vi "Stepper -- V5.vi"() -> ()   [LabVIEW 2018]
doc: "Use this template to build a producer/consumer design pattern with events to produce queue items. Use this design pattern instead of the User Interface Event Handler pattern for user interfaces when you want to execute code asynchronously in response to an event without slowing the user interface responsiveness."
uses:
  stepper motor state.ctl
  cursor range mode.ctl
  motor type.ctl
  stepper graphics action.ctl
  stepper driver action.ctl
  stepper progress monitor message.ctl
  talkto async routine action.ctl
  stepper graphics internal state.ctl
  stepper graphics internal event.ctl
  publisher action.ctl
  slider action.ctl
  stepper driver -- BLM.vi
  stepper driver -- arduino.vi
  stepper driver -- IMS.vi
panel:
  in  "Tab Control":enum32{"main", "init&stuff", "ignore", "calc"}(tab)
  in  "cur step":dbl(slide) scale=0.0..16500.0 scale format="%#.0f"
  in  "set step !":dbl(slide)=6549.0 min=0.0 max=16000.0 step=1.0 scale=0.0..16500.0
  in  "set angle!":dbl(slide)=-33.45836363636363 scale=-117.31239621859328..107.97695874136122
  in  "Stop!":bool
  in  "Go!":bool
  in  "check!":bool
  in  "stepper state":T1=enum."stopped"
  in  "XY Graph":cluster{dbl[], dbl[]}[](graph)=[{[-0.25028600695262626, -0.18003028570276625, -0.10977456445290623, -0.03951884320304622, 0.030736878046813798, 0.10099259929667381, 0.17124832054653383, 0.24150404179639384, 0.31175976304625386, 0.38201548429611387, 0.4522712055459739, 0.5225269267958339, 0.5927826480456939, 0.6630383692955539, 0.733294090545414, 0.803549811795274, 0.873805533045134, 0.944061254294994, 1.014316975544854, 1.084572696794714], [0.16539925853434134, 0.11897139648961394, 0.07254353444488655, 0.026115672400159162, -0.02031218964456824, -0.06674005168929564, -0.11316791373402302, -0.15959577577875045, -0.20602363782347782, -0.2524514998682052, -0.29887936191293263, -0.34530722395766, -0.3917350860023874, -0.43816294804711475, -0.48459081009184224, -0.5310186721365696, -0.577446534181297, -0.6238743962260244, -0.6703022582707517, -0.7167301203154792]}, {[0.14084146883576712, 0.11119063329139509, 0.08153979774702305, 0.05188896220265103, 0.022238126658278998, -0.007412708886093022, -0.037063544430465056, -0.06671437997483709, -0.09636521551920912, -0.12601605106358113, -0.15566688660795316, -0.1853177221523252, -0.21496855769669723, -0.24461939324106927, -0.2742702287854413, -0.30392106432981336, -0.33357189987418534, -0.36322273541855743, -0.3928735709629294, -0.4225244065073015], [0.26488427785767804, 0.20911916672974581, 0.1533540556018136, 0.09758894447388133, 0.04182383334594911, -0.013941277781983119, -0.06970638890991537, -0.12547150003784757, -0.18123661116577983, -0.23700172229371202, -0.2927668334216443, -0.34853194454957653, -0.4042970556775088, -0.46006216680544104, -0.5158272779333732, -0.5715923890613055, -0.6273575001892377, -0.68312261131717, -0.738887722445102, -0.7946528335730343]}, {[1.0, 0.9980267284282716, 0.9921147013144779, 0.9822872507286887, 0.9685831611286311, 0.9510565162951535, 0.9297764858882513, 0.9048270524660195, 0.8763066800438636, 0.8443279255020151, 0.8090169943749475, 0.7705132427757891, 0.7289686274214116, 0.6845471059286886, 0.6374239897486896, 0.587785252292473, 0.5358267949789965, 0.48175367410171516, 0.42577929156507266, 0.36812455268467786, 0.30901699437494745, 0.24868988716485474, 0.18738131458572452, 0.12533323356430426, 0.0627905195293133, -1.6081428723391245e-16, -0.0627905195293134, -0.12533323356430437, -0.18738131458572482, -0.24868988716485485, -0.30901699437494756, -0.368124552684678, -0.4257792915650727, -0.48175367410171543, -0.5358267949789969, -0.587785252292473, -0.6374239897486897, -0.6845471059286887, -0.7289686274214117, -0.7705132427757894, -0.8090169943749473, -0.8443279255020151, -0.8763066800438636, -0.9048270524660196, -0.9297764858882515, -0.9510565162951536, -0.9685831611286311, -0.9822872507286887, -0.9921147013144779, -0.9980267284282716, -1.0, -0.9980267284282716, -0.9921147013144779, -0.9822872507286886, -0.9685831611286311, -0.9510565162951535, -0.9297764858882512, -0.9048270524660195, -0.8763066800438635, -0.844327925502015, -0.8090169943749472, -0.770513242775789, -0.7289686274214116, -0.6845471059286886, -0.6374239897486895, -0.5877852522924732, -0.5358267949789963, -0.48175367410171527, -0.42577929156507216, -0.3681245526846778, -0.30901699437494756, -0.24868988716485443, -0.18738131458572463, -0.12533323356430373, -0.06279051952931321, -1.836909530733566e-16, 0.06279051952931372, 0.12533323356430423, 0.18738131458572513, 0.24868988716485493, 0.30901699437494723, 0.36812455268467825, 0.4257792915650726, 0.4817536741017157, 0.5358267949789968, 0.5877852522924737, 0.63742398974869, 0.6845471059286886, 0.7289686274214119, 0.7705132427757894, 0.8090169943749478, 0.8443279255020153, 0.8763066800438636, 0.9048270524660197, 0.9297764858882515, 0.9510565162951538, 0.9685831611286312, 0.9822872507286887, 0.9921147013144779, 0.9980267284282716], [0.0, 0.06279051952931337, 0.12533323356430426, 0.18738131458572463, 0.2486898871648548, 0.3090169943749474, 0.368124552684678, 0.4257792915650727, 0.4817536741017153, 0.5358267949789967, 0.5877852522924731, 0.6374239897486897, 0.6845471059286887, 0.7289686274214116, 0.7705132427757893, 0.8090169943749475, 0.8443279255020151, 0.8763066800438637, 0.9048270524660196, 0.9297764858882515, 0.9510565162951535, 0.9685831611286311, 0.9822872507286887, 0.9921147013144779, 0.9980267284282716, 1.0, 0.9980267284282716, 0.9921147013144778, 0.9822872507286886, 0.9685831611286311, 0.9510565162951535, 0.9297764858882513, 0.9048270524660195, 0.8763066800438635, 0.844327925502015, 0.8090169943749475, 0.7705132427757893, 0.7289686274214114, 0.6845471059286885, 0.6374239897486895, 0.5877852522924732, 0.5358267949789967, 0.4817536741017152, 0.4257792915650725, 0.36812455268467775, 0.3090169943749471, 0.24868988716485482, 0.18738131458572457, 0.1253332335643041, 0.06279051952931314, -3.216285744678249e-16, -0.06279051952931335, -0.12533323356430429, -0.18738131458572477, -0.24868988716485502, -0.30901699437494773, -0.3681245526846783, -0.42577929156507266, -0.4817536741017154, -0.5358267949789968, -0.5877852522924734, -0.63742398974869, -0.6845471059286887, -0.7289686274214116, -0.7705132427757894, -0.8090169943749473, -0.8443279255020153, -0.8763066800438636, -0.9048270524660198, -0.9297764858882515, -0.9510565162951535, -0.9685831611286312, -0.9822872507286887, -0.9921147013144779, -0.9980267284282716, -1.0, -0.9980267284282716, -0.9921147013144779, -0.9822872507286886, -0.9685831611286311, -0.9510565162951536, -0.9297764858882512, -0.9048270524660196, -0.8763066800438634, -0.844327925502015, -0.809016994374947, -0.770513242775789, -0.7289686274214116, -0.6845471059286883, -0.6374239897486896, -0.5877852522924726, -0.5358267949789963, -0.4817536741017153, -0.4257792915650722, -0.36812455268467786, -0.3090169943749468, -0.2486898871648545, -0.18738131458572468, -0.1253332335643038, -0.06279051952931326]}, {[0.1, 0.09980267284282716, 0.0992114701314478, 0.09822872507286887, 0.09685831611286312, 0.09510565162951537, 0.09297764858882515, 0.09048270524660196, 0.08763066800438636, 0.08443279255020152, 0.08090169943749474, 0.07705132427757892, 0.07289686274214115, 0.06845471059286887, 0.06374239897486897, 0.05877852522924731, 0.05358267949789966, 0.04817536741017152, 0.042577929156507266, 0.03681245526846779, 0.03090169943749475, 0.024868988716485477, 0.018738131458572452, 0.012533323356430426, 0.00627905195293133, -1.6081428723391246e-17, -0.0062790519529313405, -0.012533323356430436, -0.018738131458572484, -0.024868988716485487, -0.030901699437494757, -0.0368124552684678, -0.04257792915650727, -0.048175367410171546, -0.05358267949789969, -0.05877852522924731, -0.06374239897486897, -0.06845471059286888, -0.07289686274214117, -0.07705132427757895, -0.08090169943749474, -0.08443279255020152, -0.08763066800438636, -0.09048270524660197, -0.09297764858882515, -0.09510565162951537, -0.09685831611286312, -0.09822872507286888, -0.0992114701314478, -0.09980267284282716, -0.1, -0.09980267284282716, -0.0992114701314478, -0.09822872507286887, -0.09685831611286311, -0.09510565162951536, -0.09297764858882514, -0.09048270524660196, -0.08763066800438636, -0.0844327925502015, -0.08090169943749473, -0.07705132427757891, -0.07289686274214116, -0.06845471059286887, -0.06374239897486896, -0.05877852522924733, -0.05358267949789963, -0.04817536741017153, -0.04257792915650722, -0.036812455268467784, -0.03090169943749476, -0.024868988716485445, -0.018738131458572463, -0.012533323356430372, -0.0062790519529313206, -1.836909530733566e-17, 0.006279051952931373, 0.012533323356430424, 0.018738131458572515, 0.024868988716485498, 0.030901699437494726, 0.03681245526846783, 0.042577929156507266, 0.048175367410171574, 0.053582679497899674, 0.05877852522924737, 0.063742398974869, 0.06845471059286887, 0.07289686274214119, 0.07705132427757894, 0.08090169943749478, 0.08443279255020153, 0.08763066800438636, 0.09048270524660197, 0.09297764858882515, 0.09510565162951538, 0.09685831611286312, 0.09822872507286887, 0.0992114701314478, 0.09980267284282716], [0.0, 0.006279051952931338, 0.012533323356430426, 0.018738131458572466, 0.02486898871648548, 0.030901699437494743, 0.0368124552684678, 0.04257792915650727, 0.04817536741017153, 0.05358267949789967, 0.058778525229247314, 0.06374239897486898, 0.06845471059286887, 0.07289686274214116, 0.07705132427757894, 0.08090169943749476, 0.08443279255020152, 0.08763066800438638, 0.09048270524660196, 0.09297764858882515, 0.09510565162951536, 0.09685831611286312, 0.09822872507286888, 0.0992114701314478, 0.09980267284282716, 0.1, 0.09980267284282716, 0.0992114701314478, 0.09822872507286887, 0.09685831611286312, 0.09510565162951536, 0.09297764858882515, 0.09048270524660196, 0.08763066800438636, 0.0844327925502015, 0.08090169943749476, 0.07705132427757892, 0.07289686274214115, 0.06845471059286885, 0.06374239897486896, 0.05877852522924732, 0.05358267949789967, 0.048175367410171525, 0.04257792915650725, 0.03681245526846778, 0.030901699437494712, 0.024868988716485484, 0.01873813145857246, 0.01253332335643041, 0.0062790519529313145, -3.216285744678249e-17, -0.0062790519529313344, -0.012533323356430431, -0.018738131458572477, -0.0248689887164855, -0.030901699437494774, -0.03681245526846783, -0.04257792915650727, -0.04817536741017154, -0.05358267949789968, -0.05877852522924734, -0.06374239897486901, -0.06845471059286887, -0.07289686274214116, -0.07705132427757894, -0.08090169943749474, -0.08443279255020153, -0.08763066800438636, -0.09048270524660199, -0.09297764858882515, -0.09510565162951536, -0.09685831611286312, -0.09822872507286888, -0.0992114701314478, -0.09980267284282716, -0.1, -0.09980267284282716, -0.0992114701314478, -0.09822872507286887, -0.09685831611286311, -0.09510565162951537, -0.09297764858882514, -0.09048270524660196, -0.08763066800438633, -0.0844327925502015, -0.0809016994374947, -0.07705132427757891, -0.07289686274214116, -0.06845471059286884, -0.06374239897486897, -0.058778525229247265, -0.05358267949789964, -0.04817536741017153, -0.042577929156507224, -0.036812455268467784, -0.03090169943749468, -0.024868988716485452, -0.01873813145857247, -0.012533323356430379, -0.006279051952931327]}, {[-1.7, -1.7, -1.7, -1.7, -1.7, -1.7, -1.7, -1.7, -1.7, -1.7, -1.7, -1.7, -1.7, -1.7, -1.7, -1.7, -1.7, -1.7, -1.7, -1.7, -1.7, -1.6105263157894736, -1.5210526315789474, -1.431578947368421, -1.3421052631578947, -1.2526315789473683, -1.163157894736842, -1.0736842105263158, -0.9842105263157894, -0.894736842105263, -0.8052631578947368, -0.7157894736842105, -0.6263157894736842, -0.5368421052631578, -0.44736842105263164, -0.35789473684210527, -0.2684210526315789, -0.17894736842105252, -0.08947368421052615, 0.0, 0.0, 0.08947368421052632, 0.17894736842105263, 0.26842105263157895, 0.35789473684210527, 0.4473684210526316, 0.5368421052631579, 0.6263157894736842, 0.7157894736842105, 0.8052631578947369, 0.8947368421052632, 0.9842105263157894, 1.0736842105263158, 1.1631578947368422, 1.2526315789473683, 1.3421052631578947, 1.431578947368421, 1.5210526315789474, 1.6105263157894738, 1.7, 1.7, 1.7, 1.7, 1.7, 1.7, 1.7, 1.7, 1.7, 1.7, 1.7, 1.7, 1.7, 1.7, 1.7, 1.7, 1.7, 1.7, 1.7, 1.7, 1.7], [1.9, 1.7210526315789472, 1.5421052631578946, 1.3631578947368421, 1.1842105263157894, 1.0052631578947366, 0.8263157894736841, 0.6473684210526316, 0.46842105263157885, 0.2894736842105261, 0.11052631578947358, -0.06842105263157894, -0.24736842105263168, -0.4263157894736844, -0.6052631578947367, -0.7842105263157895, -0.9631578947368422, -1.142105263157895, -1.3210526315789477, -1.5, -1.5, -1.5257894736842106, -1.551578947368421, -1.5773684210526315, -1.6031578947368421, -1.6289473684210527, -1.654736842105263, -1.6805263157894736, -1.7063157894736842, -1.7321052631578948, -1.7578947368421052, -1.7836842105263158, -1.8094736842105263, -1.8352631578947367, -1.8610526315789473, -1.8868421052631579, -1.9126315789473685, -1.938421052631579, -1.9642105263157894, -1.99, -1.9900000000000002, -1.9642105263157896, -1.9384210526315793, -1.9126315789473687, -1.886842105263158, -1.8610526315789475, -1.8352631578947372, -1.8094736842105266, -1.783684210526316, -1.7578947368421054, -1.732105263157895, -1.7063157894736845, -1.6805263157894739, -1.6547368421052635, -1.628947368421053, -1.6031578947368423, -1.5773684210526318, -1.5515789473684212, -1.5257894736842108, -1.5000000000000002, -1.5, -1.3210526315789473, -1.1421052631578947, -0.9631578947368421, -0.7842105263157895, -0.6052631578947368, -0.4263157894736842, -0.24736842105263168, -0.06842105263157894, 0.1105263157894738, 0.2894736842105263, 0.46842105263157885, 0.6473684210526316, 0.8263157894736843, 1.0052631578947366, 1.1842105263157894, 1.3631578947368421, 1.5421052631578949, 1.7210526315789476, 1.9]}, {[-0.08715574274765822, -0.08899060048971419, -0.09082545823177014, -0.09266031597382611, -0.09449517371588206, -0.09633003145793803, -0.098164889199994, -0.09999974694204995, -0.10183460468410592, -0.10366946242616187, -0.10550432016821784, -0.10733917791027381, -0.10917403565232978, -0.11100889339438573, -0.1128437511364417, -0.11467860887849765, -0.11651346662055362, -0.11834832436260959, -0.12018318210466554, -0.12201803984672151], [0.9961946980917454, 1.0171672180515716, 1.038139738011398, 1.059112257971224, 1.0800847779310503, 1.1010572978908766, 1.1220298178507027, 1.143002337810529, 1.1639748577703553, 1.1849473777301813, 1.2059198976900076, 1.2268924176498337, 1.24786493760966, 1.2688374575694863, 1.2898099775293124, 1.3107824974891387, 1.3317550174489647, 1.352727537408791, 1.3737000573686173, 1.3946725773284436]}, {[-0.46947156278589053, -0.47935517463401456, -0.48923878648213853, -0.49912239833026256, -0.5090060101783865, -0.5188896220265106, -0.5287732338746346, -0.5386568457227586, -0.5485404575708825, -0.5584240694190066, -0.5683076812671306, -0.5781912931152546, -0.5880749049633787, -0.5979585168115026, -0.6078421286596266, -0.6177257405077506, -0.6276093523558747, -0.6374929642039986, -0.6473765760521226, -0.6572601879002467], [-0.882947592858927, -0.9015359632349044, -0.9201243336108818, -0.9387127039868592, -0.9573010743628366, -0.975889444738814, -0.9944778151147914, -1.0130661854907688, -1.0316545558667463, -1.0502429262427238, -1.068831296618701, -1.0874196669946785, -1.1060080373706558, -1.1245964077466333, -1.1431847781226105, -1.161773148498588, -1.1803615188745655, -1.1989498892505428, -1.2175382596265203, -1.2361266300024978]}, {[-0.6572601879002467, -0.6108630096264345, -0.5636217044296241, -0.515601553161604, -0.46686891293009347, -0.41749112540253713, -0.3675364237493727, -0.31707383835536895, -0.26617310142932604, -0.21490455064395006, -0.1633390319390661, -0.11154780162247316, -0.05960242790373095, -0.007574691996942432, 0.044463511070809286, 0.09644027180829284, 0.1482837656289526, 0.19992235210240325, 0.25128467395144666, 0.3022997556578122, 0.35289710154035936, 0.4030067931702119, 0.45255958598821155, 0.5014870049911768, 0.5497214393547454, 0.5971962358620418, 0.643845791009066, 0.6896056416595259, 0.7344125541238411, 0.7782046115392272, 0.8209212994301052, 0.8625035893306137, 0.9028940203536602, 0.9420367785938017, 0.979877774254226, 1.0163647163912568, 1.0514471851730987, 1.0850767015529643, 1.1172067942603134, 1.1477930640176235, 1.176793244893958, 1.204167262710551, 1.2298772904176951, 1.2538878003664136, 1.276165613402685, 1.2966799447163748, 1.3154024463815224, 1.3323072465291936, 1.3473709850987734, 1.360572846118289, 1.3718945864691614, 1.3813205610956336, 1.3888377446240419, 1.3944357493620536, 1.3981068396529994, 1.3998459425654655, 1.399650654903371, 1.3975212465268496, 1.3934606599793398, 1.3874745064214027, 1.379571057876886, 1.3697612358021491, 1.3580585959941422, 1.3444793098581995, 1.3290421420614258, 1.3117684246025616, 1.2926820273341562, 1.2718093249777804, 1.249179160677867, 1.2248228061445314, 1.1987739184404593, 1.1710684934715725, 1.141744816245737, 1.1108434079682614, 1.078406970047275, 1.0444803250863792, 1.0091103549461014, 0.9723459359597438, 0.9342378713931556, 0.894838821241748, 0.8542032294617747, 0.8123872487364283, 0.7694486628807135, 0.7254468069923291, 0.6804424854588903, 0.6344978879348022, 0.5876765034038882, 0.5400430324465261, 0.49166329783253176, 0.4426041535633281, 0.39293339248910303, 0.34271965262860676, 0.2920323223210451, 0.24094144434113837, 0.18951761910983606, 0.1378319071344487, 0.08595573081300137, 0.033960775738508885, -0.018081108360453915, -0.07009800690598791], [-1.2361266300024978, -1.259700910323611, -1.2815344608303927, -1.301597110621156, -1.319861135930395, -1.3363012984391367, -1.3508948801507545, -1.3636217147840501, -1.374464215640223, -1.38340739990522, -1.3904389093538805, -1.3955490274272677, -1.3987306926595915, -1.3999795084361597, -1.399293749068885, -1.3966743621809423, -1.392124967397287, -1.3856518513428409, -1.3772639589552595, -1.3669728811242843, -1.3547928386747596, -1.3407406627154492, -1.3248357713808072, -1.307100142997842, -1.2875582857151542, -1.266237203636115, -1.243166359502987, -1.2183776339835501, -1.1919052816164948, -1.1637858834764583, -1.1340582966241142, -1.1027636004111705, -1.0699450397144725, -1.0356479651776527, -0.999919770542909, -0.962809827159507, -0.9243694157595043, -0.8846516555949799, -0.8437114310346835, -0.8016053157215436, -0.7583914943958356, -0.7141296824920375, -0.6688810436204844, -0.6227081050478439, -0.5756746712932125, -0.5278457359592277, -0.47928739192003167, -0.4300667399902001, -0.3802517962008339, -0.3299113978109549, -0.279115108184076, -0.22793312066139887, -0.17643616156447195, -0.12469539246134045, -0.07278231183125206, -0.020768656263793716, 0.0312736986710031, 0.08327283774461088, 0.1351569054467535, 0.18685420527963775, 0.23829329883244557, 0.2894031044991896, 0.3401129957035144, 0.39035289849470745, 0.44005338838006564, 0.48914578625979516, 0.5375622533318869, 0.5852358848358173, 0.6321008025055334, 0.6780922456039706, 0.7231466604132986, 0.7672017880572369, 0.8101967505340834, 0.8520721348415629, 0.8927700750772594, 0.9322343324011679, 0.970410372749876, 1.0072454421949844, 1.0426886398416284, 1.0766909881663722, 1.1092055006972668, 1.140187246942561, 1.1695934144783315, 1.1973833681092427, 1.2235187060206834, 1.2479633128446825, 1.2706834095662773, 1.2916476002013708, 1.310826915181573, 1.3281948513860795, 1.3437274087652615, 1.3574031235053672, 1.3692030976884975, 1.3791110254068764, 1.3871132152953265, 1.3931986094508135, 1.3973587987129157, 1.3995880342841027, 1.3998832356737676, 1.398243994955032]}]
  in  "motor selector":T2=enum."--"
  in  "Instrument Address":refnum<visa-resource-name>="ASRL3::INSTR"
  in  "set speed!":bool
  in  "speed":dbl=2.0 format="%_2f"
  in  "sync to":bool
  in  "syncto":dbl format="%_2f"
  in  "cursor mode":T3
  in  "response message":cluster{"step (fdeg)":dbl}={"step (fdeg)"=310.3875004849805}
  out "progress monitor VI":refnum<vi>
  out "cur angle":dbl(slide)=-118.0 scale=-117.31239621859328..107.97695874136122 scale format="%#.0f"
  in  "angle aux":dbl(slide)=86.23585875899897 scale=0.0..90.0 scale format="%#.0f"
  in  "step aux":dbl(slide)=16500.0 scale=0.0..8886.0 scale format="%#.0f"
  in  "dir":u16(ring)
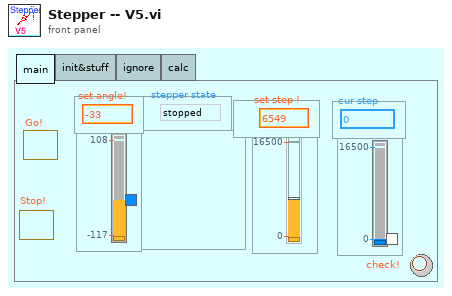
[diagram p1: front panel]
types:
  T1 = typedef "stepper motor state.ctl" = enum16{"moving", "stopped"}
  T2 = typedef "motor type.ctl" = enum16{"IMS", "arduino C&A", "BLM", "--"}
  T3 = typedef "cursor range mode.ctl" = enum16{"change angle", "lock", "extend"}
  T4 = typedef "stepper graphics action.ctl" = enum16{"--update circle", "set step slider moves", "cursor moves", "current step changed", "init", "void", "--draw current line", "--draw set line", "--move current step slider", "--move set step slider", "--draw limit lines", "check", "--move set angle slider", "--move current angle slider", "set angle slider moves", "--move center cursor", "set set step", "set current step", "read", "--move limit-cursors", "cursor release", "current step moves"}
  T5 = typedef "stepper driver action.ctl" = enum16{"go", "void", "stop", "check", "init", "sync", "set", "set speed", "--check status", "--check value", "--handshake"}
  T6 = typedef "stepper graphics internal event.ctl" = enum16{"set slider moves", "update scale", "exit", "current positon changed", "stop", "go", "set speed", "set to zero", "sync", "check"}
  T7 = typedef "stepper graphics internal state.ctl" = cluster{"set pos slider":refnum<vi>, "cur angle slider":refnum<vi>, "XY Graph":refnum<vi>, "set angle":dbl, "current angle":dbl, "set angle slider":refnum<vi>, "current pos... slider":refnum<vi>, "current pos":dbl, "set pos":dbl}
  T8 = typedef "talkto async routine action.ctl" = enum16{"stop", "check"}
  T9 = typedef "stepper progress monitor message.ctl" = cluster{"current position":dbl, "stepper motor state OUT":T1}
  T10 = typedef "publisher action.ctl" = enum16{"set", "get", "init", "check"}
  T11 = typedef "slider action.ctl" = enum16{"check", "copy range -- keep value", "set from value", "set from ratio", "set from slider", "read using other slider", "set lower limit", "set upper limit", "set lower from slider", "set upper from slider", "copy range -- keep ratio", "set using other slider -- no check"}
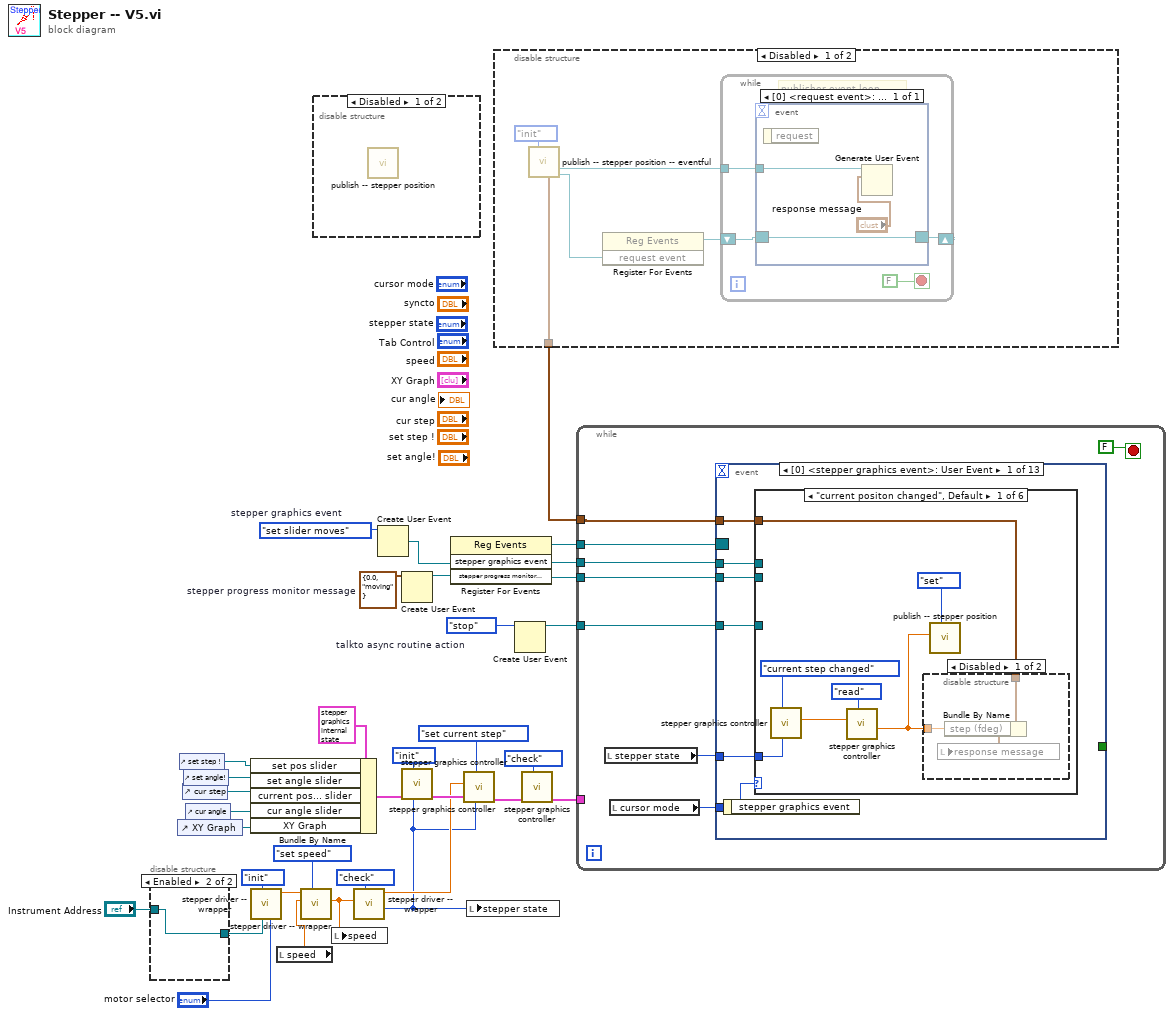
[diagram p0: block diagram]
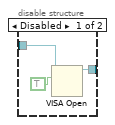
[diagram p2: hidden frame]
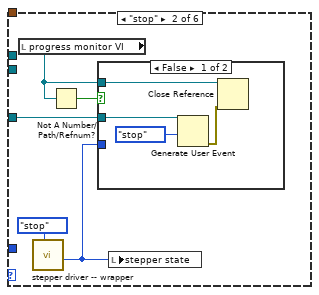
[diagram p6: hidden frame]
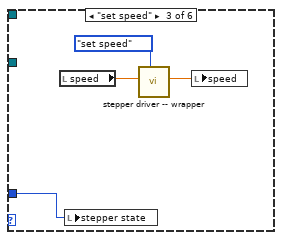
[diagram p8: hidden frame]
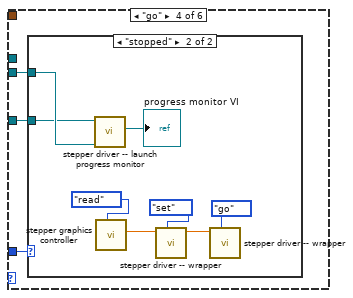
[diagram p9: hidden frame]
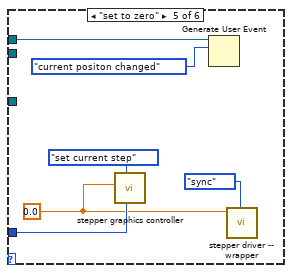
[diagram p11: hidden frame]
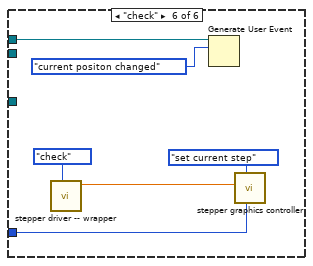
[diagram p12: hidden frame]
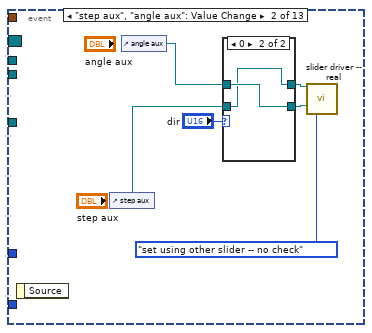
[diagram p13: hidden frame]
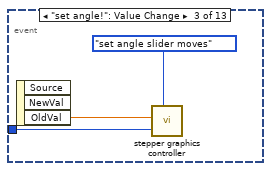
[diagram p15: hidden frame]
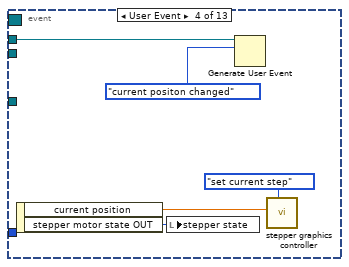
[diagram p16: hidden frame]
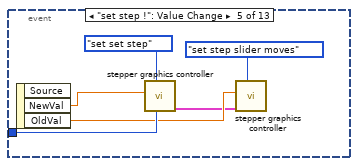
[diagram p17: hidden frame]
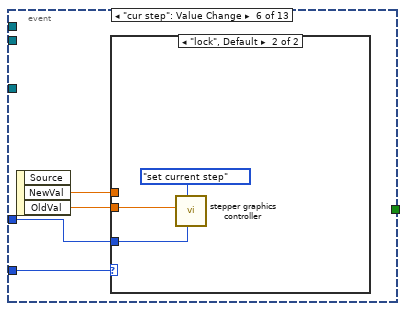
[diagram p18: hidden frame]
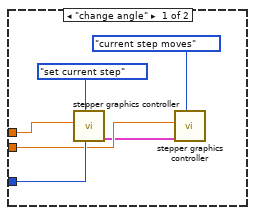
[diagram p19: hidden frame]
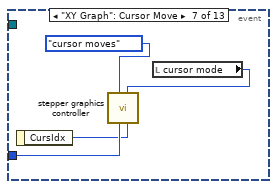
[diagram p20: hidden frame]
diagram:
  w15 = stepper_graphics_internal_event."set slider moves"  # stepper graphics event
  w25 = talkto_async_routine_action."stop"  # talkto async routine action
  w27 = T9 {"current position"=0.0, "stepper motor state OUT"=enum."moving"}  # stepper progress monitor message
  n1 = disable-structure shown="Enabled" {
    disable-tunnel: "Instrument Address" -> [w34 w36]
    disable-tunnel: [w33 w36] -> w14
    frame Disabled {
      n2 = VISA Open(duplicate session (F)=TRUE, VISA resource name=w34) -> (VISA resource name=w33:refnum<visa-resource-name>)  [unwired: 3 in, 1 out]
    }
    frame Enabled {
    }
  }
  n3 = control-ref of="XY Graph"() -> (w18:refnum<vi>)
  n4 = control-ref of="set step !"() -> (w22:refnum<vi>)
  n5 = control-ref of="cur step"() -> (w20:refnum<vi>)
  n6 = control-ref of="set angle!"() -> (w21:refnum<vi>)
  n7 = control-ref of="cur angle"() -> (w19:refnum<vi>)
  n8 = Bundle By Name(cluster=T7 {"set pos slider"=refnum, "cur angle slider"=refnum, "XY Graph"=refnum, "set angle"=0.0, "current angle"=0.0, "set angle slider"=refnum, "current pos... slider"=refnum, "current pos"=0.0, "set pos"=0.0} ("stepper graphics internal state"), "set pos slider"=w22, "set angle slider"=w21, "current pos... slider"=w20, "cur angle slider"=w19, "XY Graph"=w18) -> (w16:T7)
  n9 = call "stepper driver -- wrapper.vi"("motor selector"="motor selector", "Instrument Address"=w14, "stepper driver action"=stepper_driver_action."init") -> ("number OUT"=w12:dbl)  [unwired: 6 in, 2 out]
  n10 = local read "speed"() -> (w13:dbl)
  n11 = call "stepper driver -- wrapper.vi"("stepper driver action"=stepper_driver_action."set speed", "speed IN"=w13, "number IN"=w12) -> ("speed OUT"=w6:dbl)  [unwired: 6 in, 2 out]
  n12 = disable-structure shown="Disabled" {
    frame Disabled {
      n13 = call "publish -- stepper position.vi"() -> ()  [unwired: 11 in, 1 out]
    }
    frame Enabled {
    }
  }
  n14 = local write "speed"(w6) -> ()
  n15 = call "stepper driver -- wrapper.vi"("stepper driver action"=stepper_driver_action."check", "speed IN"=w6) -> ("stepper motor state OUT"=w5:T1, "number OUT"=w7:dbl)  [unwired: 7 in, 1 out]
  n16 = Create User Event(user event datatype=w15) -> (user event=w28:refnum<user-event>)  [unwired: 1 in, 1 out]
  n17 = Create User Event(user event datatype=w27) -> (user event=w26:refnum<user-event>)  [unwired: 1 in, 1 out]
  n18 = call "stepper graphics controller.vi"("stepper motor state"=w5, "stepper graphics action"=stepper_graphics_action."init", "stepper graphics internal state"=w16) -> ("stepper graphics internal state OUT"=w8:T7)  [unwired: 6 in, 2 out]
  n19 = register-events(w28, w26) -> (reference out=w31:refnum<event-registration>)  [unwired: 2 in, 1 out]
  n20 = call "stepper graphics controller.vi"("stepper motor state"=w5, "stepper graphics action"=stepper_graphics_action."set current step", "stepper graphics internal state"=w8, "value"=w7) -> ("stepper graphics internal state OUT"=w3:T7)  [unwired: 5 in, 2 out]
  n21 = local write "stepper state"(w5) -> ()
  n22 = disable-structure shown="Disabled" {
    disable-tunnel: [w37 _] -> w11
    frame Disabled {
      n23 = call "publish -- stepper position -- eventful.vi"("publisher action"=publisher_action."init") -> ("response event"=w38:refnum<user-event>, "response type"=w37:cluster{"step (fdeg)":dbl}, "request event"=w39:refnum<user-event>)  [unwired: 11 in, 1 out]
      n24 = register-events(w39) -> (reference out=w40:refnum<event-registration>)  [unwired: 2 in, 1 out]
      n25 = while {
        shift-right: [w44] -> _
        shift-left: w40 -> [w43]
        tunnel: w38 -> [w42]
        stop <- FALSE stop-if-true
        # "publisher event loop"
        n26 = event shown="[0] <request event>: User Event" {
          selector: w43 -> [w48]
          dyn-events: [w48] -> w44
          timeout: _ -> [_]
          tunnel: w42 -> [w47]
          event User Event {
            n27 = event-data() -> ()  [unwired: 1 in, 1 out]
            n28 = Generate User Event(user event=w47, event data cluster="response message") -> ()  [unwired: 2 in, 2 out]
          }
        }
      }
    }
    frame Enabled {
    }
  }
  n29 = Create User Event(user event datatype=w25) -> (user event=w24:refnum<user-event>)  [unwired: 1 in, 1 out]
  n30 = call "stepper graphics controller.vi"("stepper graphics action"=stepper_graphics_action."check", "stepper graphics internal state"=w3) -> ("stepper graphics internal state OUT"=w2:T7)  [unwired: 7 in, 2 out]
  n31 = while {
    tunnel: w31 -> [w56]
    tunnel: w28 -> [w55]
    tunnel: w26 -> [w53]
    tunnel: w24 -> [w52]
    tunnel: w11 -> [w50]
    tunnel: w2 -> [_]
    stop <- FALSE stop-if-true
    n32 = local read "stepper state"() -> (w54:T1)
    n33 = local read "cursor mode"() -> (w49:T3)
    n34 = event shown="[0] <stepper graphics event>: User Event" {
      selector: w56 -> [_ _ _ _ _ _ _ _ _ _ _ _ _]
      dyn-events: _ -> [_ _ _ _ _ _ _ _ _ _ _ _ _]
      timeout: _ -> [_ _ _ _ _ _ _ _ _ _ _ _ _]
      tunnel: w55 -> [w60 _ _ w123 _ _ _ _ w154 w158 w161 w164 w167]
      tunnel: w54 -> [w61 _ w119 _ w131 w136 w148 w151 _ _ _ _ _]
      tunnel: [_ _ _ _ _ _ _ _ "Stop!" "set speed!" "Go!" "check!" "sync to"] -> _
      tunnel: w53 -> [w59 _ _ _ _ _ _ _ _ _ _ _ _]
      tunnel: w52 -> [w58 _ _ _ _ _ _ _ _ _ _ _ _]
      tunnel: w50 -> [w57 _ _ _ _ _ _ _ _ _ _ _ _]
      tunnel: w49 -> [_ _ _ _ _ w133 _ _ _ _ _ _ _]
      event User Event {
        n35 = event-data() -> ("stepper graphics event"=w62:T6)  [unwired: 1 in]
        n36 = case shown="\"current positon changed\", Default" w62 {
          tunnel: w61 -> [w68 _ w82 w87 w101 w107]
          tunnel: w60 -> [_ _ _ _ w99 w105]
          tunnel: w59 -> [_ _ _ w88 _ _]
          tunnel: w58 -> [_ w74 _ w86 _ _]
          tunnel: w57 -> [w65 _ _ _ _ _]
          frame "current positon changed", Default {
            n37 = call "stepper graphics controller.vi"("stepper motor state"=w68, "stepper graphics action"=stepper_graphics_action."current step changed") -> ("set pos"=w66:dbl)  [unwired: 7 in, 2 out]
            n38 = call "stepper graphics controller.vi"("stepper graphics action"=stepper_graphics_action."read", "value"=w66) -> ("current pos"=w64:dbl)  [unwired: 7 in, 2 out]
            n39 = disable-structure shown="Disabled" {
              disable-tunnel: w64 -> [w72 _]
              disable-tunnel: w65 -> [w70 _]
              frame Disabled {
                n40 = Bundle By Name(cluster=w70, "step (fdeg)"=w72) -> (w71:cluster{"step (fdeg)":dbl})
                n41 = local write "response message"(w71) -> ()
              }
              frame Enabled {
              }
            }
            n42 = call "publish -- stepper position.vi"("publisher action"=publisher_action."set", "stepper pos IN"=w64) -> ()  [unwired: 9 in, 1 out]
          }
          frame "stop" {
            n43 = local read "progress monitor VI"() -> (w76:refnum<vi>)
            n44 = call "stepper driver -- wrapper.vi"("stepper driver action"=stepper_driver_action."stop") -> ("stepper motor state OUT"=w73:T1)  [unwired: 8 in, 2 out]
            n45 = Not A Number/Path/Refnum?(number/path/refnum=w76) -> (NaN/Path/Refnum?=w75:bool)
            n46 = case shown="False" w75 {
              tunnel: w76 -> [w81 _]
              tunnel: w74 -> [w80 _]
              tunnel: w73 -> [_ _]
              frame False {
                n47 = Generate User Event(user event=w80, event data cluster=talkto_async_routine_action."stop" ("event data")) -> (error out=w78:errorcluster)  [unwired: 2 in, 1 out]
                n48 = Close Reference(reference=w81, error in (no error)=w78) -> ()  [unwired: 1 out]
              }
              frame True {
              }
            }
            n49 = local write "stepper state"(w73) -> ()
          }
          frame "set speed" {
            n50 = local read "speed"() -> (w84:dbl)
            n51 = local write "stepper state"(w82) -> ()
            n52 = call "stepper driver -- wrapper.vi"("stepper driver action"=stepper_driver_action."set speed", "speed IN"=w84) -> ("speed OUT"=w83:dbl)  [unwired: 7 in, 2 out]
            n53 = local write "speed"(w83) -> ()
          }
          frame "go" {
            n54 = case shown="\"stopped\"" w87 {
              tunnel: w88 -> [_ w94]
              tunnel: w86 -> [_ w93]
              frame "moving", Default {
              }
              frame "stopped" {
                n55 = call "stepper driver -- launch progress monitor.vi"("talkback  user event"=w94, "talkto user event"=w93) -> ("reference out"=→"progress monitor VI":refnum<vi>)  [unwired: 9 in]
                n56 = call "stepper graphics controller.vi"("stepper graphics action"=stepper_graphics_action."read") -> ("set pos"=w91:dbl)  [unwired: 8 in, 2 out]
                n57 = call "stepper driver -- wrapper.vi"("stepper driver action"=stepper_driver_action."set", "number IN"=w91) -> ("number OUT"=w90:dbl)  [unwired: 7 in, 2 out]
                n58 = call "stepper driver -- wrapper.vi"("stepper driver action"=stepper_driver_action."go", "number IN"=w90) -> ()  [unwired: 7 in, 3 out]
              }
            }
          }
          frame "set to zero" {
            w97 = 0.0 ("value")
            n59 = call "stepper graphics controller.vi"("stepper motor state"=w101, "stepper graphics action"=stepper_graphics_action."set current step", "value"=w97) -> ()  [unwired: 6 in, 3 out]
            n60 = Generate User Event(user event=w99, event data cluster=stepper_graphics_internal_event."current positon changed" ("event data")) -> ()  [unwired: 2 in, 2 out]
            n61 = call "stepper driver -- wrapper.vi"("stepper driver action"=stepper_driver_action."sync", "number IN"=w97) -> ()  [unwired: 7 in, 3 out]
          }
          frame "check" {
            n62 = call "stepper driver -- wrapper.vi"("stepper driver action"=stepper_driver_action."check") -> ("number OUT"=w104:dbl)  [unwired: 8 in, 2 out]
            n63 = Generate User Event(user event=w105, event data cluster=stepper_graphics_internal_event."current positon changed" ("event data")) -> ()  [unwired: 2 in, 2 out]
            n64 = call "stepper graphics controller.vi"("stepper motor state"=w107, "stepper graphics action"=stepper_graphics_action."set current step", "value"=w104) -> ()  [unwired: 6 in, 3 out]
          }
        }
      }
      event "step aux", "angle aux": Value Change {
        n65 = event-data() -> ()  [unwired: 1 in, 1 out]
        n66 = control-ref of="step aux"() -> (w110:refnum<vi>)
        n67 = control-ref of="angle aux"() -> (w112:refnum<vi>)
        n68 = case shown="0" "dir" {
          tunnel: [w116 w117] -> w113
          tunnel: w112 -> [w116 w118]
          tunnel: [w115 w118] -> w111
          tunnel: w110 -> [w115 w117]
          frame 1, Default {
          }
          frame 0 {
          }
        }
        n69 = call "slider driver -- real.vi"("slider in"=w113, "slider action"=slider_action."set using other slider -- no check", "slider from"=w111) -> ()  [unwired: 8 in, 5 out]
      }
      event "set angle!": Value Change {
        n70 = event-data() -> ("OldVal"=w121:dbl)  [unwired: 1 in, 2 out]
        n71 = call "stepper graphics controller.vi"("stepper motor state"=w119, "stepper graphics action"=stepper_graphics_action."set angle slider moves", "value"=w121) -> ()  [unwired: 6 in, 3 out]
      }
      event User Event {
        n72 = event-data() -> ("current position"=w125:dbl, "stepper motor state OUT"=w124:T1)  [unwired: 1 in]
        n73 = local write "stepper state"(w124) -> ()
        n74 = Generate User Event(user event=w123, event data cluster=stepper_graphics_internal_event."current positon changed" ("event data")) -> ()  [unwired: 2 in, 2 out]
        n75 = call "stepper graphics controller.vi"("stepper graphics action"=stepper_graphics_action."set current step", "value"=w125) -> ()  [unwired: 7 in, 3 out]
      }
      event "set step !": Value Change {
        n76 = event-data() -> ("NewVal"=w129:dbl, "OldVal"=w128:dbl)  [unwired: 1 in, 1 out]
        n77 = call "stepper graphics controller.vi"("stepper motor state"=w131, "stepper graphics action"=stepper_graphics_action."set set step", "value"=w129) -> ("stepper graphics internal state OUT"=w127:T7)  [unwired: 6 in, 2 out]
        n78 = call "stepper graphics controller.vi"("stepper graphics action"=stepper_graphics_action."set step slider moves", "stepper graphics internal state"=w127, "value"=w128) -> ()  [unwired: 6 in, 3 out]
      }
      event "cur step": Value Change {
        n79 = event-data() -> ("NewVal"=w135:dbl, "OldVal"=w134:dbl)  [unwired: 1 in, 1 out]
        n80 = case shown="\"lock\", Default" w133 {
          tunnel: w136 -> [w141 w144]
          tunnel: w135 -> [w139 _]
          tunnel: w134 -> [w138 w143]
          frame "change angle" {
            n81 = call "stepper graphics controller.vi"("stepper motor state"=w141, "stepper graphics action"=stepper_graphics_action."set current step", "value"=w139) -> ("stepper graphics internal state OUT"=w137:T7)  [unwired: 6 in, 2 out]
            n82 = call "stepper graphics controller.vi"("stepper graphics action"=stepper_graphics_action."current step moves", "stepper graphics internal state"=w137, "value"=w138) -> ()  [unwired: 6 in, 3 out]
          }
          frame "lock", Default {
            n83 = call "stepper graphics controller.vi"("stepper motor state"=w144, "stepper graphics action"=stepper_graphics_action."set current step", "value"=w143) -> ()  [unwired: 6 in, 3 out]
          }
        }
      }
      event "XY Graph": Cursor Move {
        n84 = event-data() -> ("CursIdx"=w147:i32)  [unwired: 1 in]
        n85 = local read "cursor mode"() -> (w146:T3)
        n86 = call "stepper graphics controller.vi"("cursor index"=w147, "cursor range mode"=w146, "stepper motor state"=w148, "stepper graphics action"=stepper_graphics_action."cursor moves") -> ()  [unwired: 5 in, 3 out]
      }
      event "XY Graph": Cursor Release {
        n87 = event-data() -> ("CursIdx"=w150:i32)  [unwired: 1 in]
        n88 = call "stepper graphics controller.vi"("cursor index"=w150, "stepper motor state"=w151, "stepper graphics action"=stepper_graphics_action."cursor release") -> ()  [unwired: 6 in, 3 out]
      }
      event "Stop!": Value Change {
        n89 = event-data() -> ()  [unwired: 1 in, 1 out]
        n90 = Generate User Event(user event=w154, event data cluster=stepper_graphics_internal_event."stop" ("event data")) -> ()  [unwired: 2 in, 2 out]
      }
      event "set speed!": Value Change {
        n91 = event-data() -> ()  [unwired: 1 in, 1 out]
        n92 = Generate User Event(user event=w158, event data cluster=stepper_graphics_internal_event."set speed" ("event data")) -> ()  [unwired: 2 in, 2 out]
      }
      event "Go!": Value Change {
        n93 = event-data() -> ()  [unwired: 1 in, 1 out]
        n94 = Generate User Event(user event=w161, event data cluster=stepper_graphics_internal_event."go" ("event data")) -> ()  [unwired: 2 in, 2 out]
      }
      event "check!": Value Change {
        n95 = event-data() -> ()  [unwired: 1 in, 1 out]
        n96 = Generate User Event(user event=w164, event data cluster=stepper_graphics_internal_event."check" ("event data")) -> ()  [unwired: 2 in, 2 out]
      }
      event "sync to": Value Change {
        n97 = event-data() -> ()  [unwired: 1 in, 1 out]
        n98 = Generate User Event(user event=w167, event data cluster=stepper_graphics_internal_event."set to zero" ("event data")) -> ()  [unwired: 2 in, 2 out]
      }
    }
  }
